vi "Init Match.vi"(4 "Not found":refnum<class "CConfig Query.lvclass">, 5 "Regex [F]":bool, 6 "Found":refnum<class "CConfig Query.lvclass">, 7 "Data [name]":T1=enum."name", 8 "error in (no error)":errorcluster, 9 "Invert [F]":bool, 10 "Data":string) -> (0 "error out":errorcluster, 3 "Find First Query out":refnum<class "Loop Query.lvclass">)   [LabVIEW 2013, in "Match Query.lvclass"]
doc: "Copyright 2018, Carya Automatisering, Wiebe Walstra."
uses:
  Match Query.lvclass
  Loop Query.lvclass
  CConfig Query.lvclass
  Data.ctl
  Match Query.lvclass/Match Query.ctl
  CConfig Object.lvclass
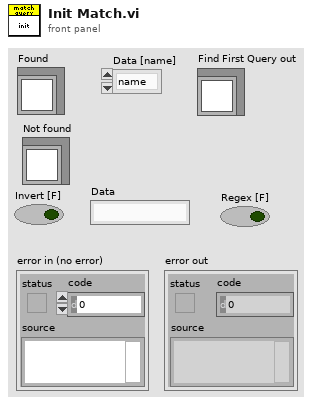
[diagram p1: front panel]
types:
  T1 = typedef "CConfig Object.lvclass/Data.ctl" = enum16{"pre", "name", "middle", "value", "post", "newline", "persistant", "tagged", "type"}
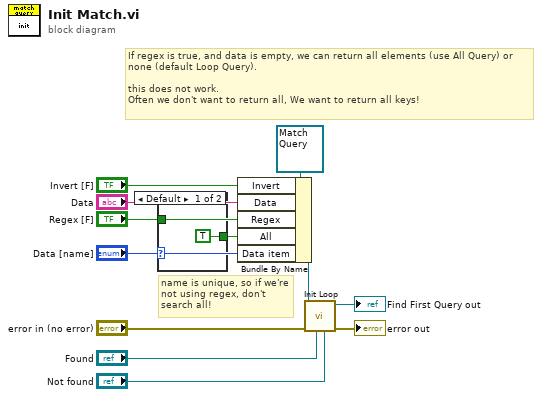
[diagram p0: block diagram]
diagram:
  # "name is unique, so if we're not using regex, don't search all!"
  # "If regex is true, and data is empty, we can return all elements (use All Query) or none (default Loop Query).\n\nthis does not work.\nOften we don't want to return all, We want to return all keys!"
  n1 = case shown="Default" "Data [name]" {
    tunnel: "Regex [F]" -> [_ w14]
    tunnel: [TRUE ("Regex [F]") w14] -> w1
    frame Default {
    }
    frame "name" {
    }
  }
  n2 = Bundle By Name(cluster=refnum<class "Match Query.lvclass"> refnum ("Find First Query in"), "Invert"="Invert [F]", "Data"="Data", "Regex"="Regex [F]", "All"=w1, "Data item"="Data [name]") -> (w2:refnum<class "Match Query.lvclass">)
  n3 = call "Init Loop.vi"("Not found"="Not found", "Found"="Found", "error in (no error)"="error in (no error)", "Loop Query"=w2) -> ("error out"=→"error out":errorcluster, "Loop Query"=→"Find First Query out":refnum<class "Match Query.lvclass">)  [unwired: 6 in]
